vi "GenerationProducerConsumer.vi"() -> ()   [LabVIEW 2022 SP3, in "Generation.lvlib"]
uses:
  Generation.lvlib
  Message.ctl
  FrameProperties.ctl
  <vilib>/platform/TimedLoop/XDataNode/XDataNode.xnode
  <vilib>/Platform/TimedLoop/XDataNode/timing_clust.ctl
  <vilib>/Platform/TimedLoop/XDataNode/XDNodeRunTimeDep.lvlib
  <vilib>/Platform/TimedLoop/XDataNode/wakeup.ctl
  <vilib>/Platform/TimedLoop/XDataNode/nitl_modes.ctl
  <vilib>/DAQmx/write.llb/DAQmx Write (Analog Wfm 1Chan NSamp).vi
panel:
  in  "Cluster":T1={"data"={"t0"=timestamp(0 s since 1904-01-01), "dt"=0.0, "Y"=[]}, "Output task"="", "error in"={"status"=FALSE, "code"=0, "source"=""}}
  in  "queue out":refnum<queue>
  out "task out":refnum<k21>
  out "error out":errorcluster
  out "Generation Duration(ns)":i64
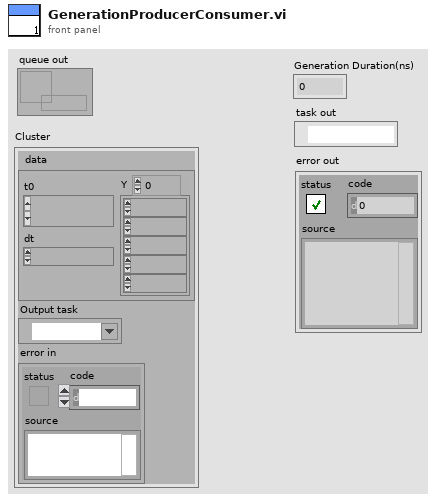
[diagram p1: front panel]
types:
  T1 = cluster{"data":waveform(dbl), "Output task":refnum<k21>, "error in":errorcluster}
  T2 = typedef "XDNodeRunTimeDep.lvlib/timing_clust.ctl" = cluster{"Expected End [f-1]":u64, "Actual End [f-1]":u64, "Finished Late? [f-1]":bool, "Expected End [i-1]":u64, "Actual End [i-1]":u64, "Finished Late? [i-1]":bool, "Expected Start [i]":u64, "Actual Start [i]":u64, "Expected Start [f]":u64, "Actual Start [f]":u64, "Source Name":string, "Structure Name":string, "Period":i64, "Deadline":i64, "Offset":i64, "Start":i64, "Priority":i32, "Timeout":i32, "Mode":T3, "Wakeup Reason":T4, "Error":errorcluster, "Source Type":string, "Secondary Source Type":string, "Global End Time":u64, "Global Start Time":u64, "Frame Duration":u64, "Iteration Duration":u64, "Assigned CPU":i32, "I/O Scan Engine Mode":u32}
  T3 = typedef "XDNodeRunTimeDep.lvlib/nitl_modes.ctl" = enum32{"No Change", "Process missed periods, maintain original phase", "Discard missed periods, maintain original phase", "Process missed periods, ignore original phase", "Discard missed periods, ignore original phase"}
  T4 = typedef "XDNodeRunTimeDep.lvlib/wakeup.ctl" = enum32{"Normal", "Aborted", "Asynchronous wakeup", "Timing source error", "Timed loop error", "Timeout"}
  T5 = typedef "FrameProperties.ctl" = cluster{"Frame Duration":i64, "Actual Start [i]":i64}
  T6 = typedef "Message.ctl" = cluster{"FrameProperties":cluster{"Frame Duration":i64, "Actual Start [i]":i64}, "Data":waveform(dbl), "Identifier":enum16{"Accel", "SignalOut", "ButtonPress"}}
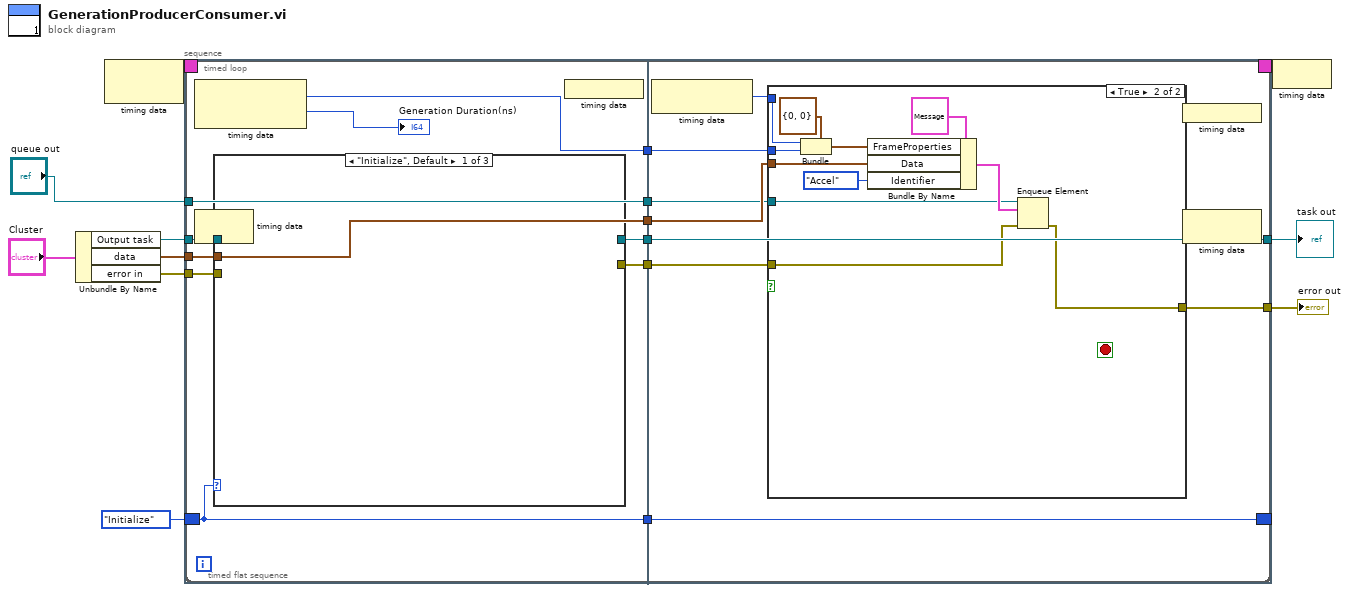
[diagram p0: block diagram]
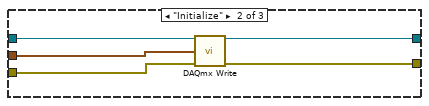
[diagram p2: hidden frame]
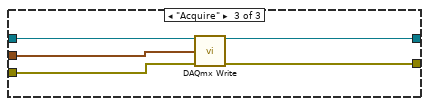
[diagram p3: hidden frame]
diagram:
  n1 = Unbundle By Name("Cluster") -> ("Output task"=w4:refnum<k21>, "data"=w3:waveform(dbl), "error in"=w2:errorcluster)
  n2 = node-c288() -> (w10:T2)  [unwired: 1 in]
  n3 = timed-loop {
    timing: w10 -> [_]
    timing-out: [_] -> w9
    tunnel: w4 -> [w18]
    tunnel: [w17] -> w7
    tunnel: "queue out" -> [w16]
    tunnel: [w15] -> w8
    tunnel: w2 -> [w14]
    tunnel: w3 -> [w13]
    shift-right: [w12] -> _
    shift-left: enum16{"Initialize", "Acquire", "Stop"}."Initialize" -> [w11]
    stop <- _ stop-if-true
    n4 = timed-sequence {
      timing: _ -> [_]
      timing-out: _ -> [_]
      tunnel: w18 -> [w32]
      tunnel: [w26] -> w17
      tunnel: w16 -> [w25]
      tunnel: [w24] -> w15
      tunnel: w14 -> [w23]
      tunnel: w13 -> [w22]
      tunnel: [w20] -> w12
      tunnel: w11 -> [w19]
      n5 = timed-flat-sequence {
        tunnel: w32 -> [w41]
        tunnel: [w39] -> w31
        tunnel: [w34] -> w30
        tunnel: [w38] -> w29
        tunnel: [w37] -> w28
        tunnel: [w36] -> w27
        tunnel: w25 -> [w38]
        tunnel: w23 -> [w35]
        tunnel: w22 -> [w34]
        tunnel: [w33] -> w21
        tunnel: w19 -> [w33]
        tunnel: w31 -> [w62]
        tunnel: w30 -> [w61]
        tunnel: w29 -> [w60]
        tunnel: w28 -> [w59]
        tunnel: w27 -> [w57]
        tunnel: [w57] -> w26
        tunnel: [w58] -> w24
        tunnel: w21 -> [w56]
        tunnel: [w56] -> w20
        frame #0 {
          n6 = node-c288() -> (w39:i64, →"Generation Duration(ns)":i64)  [unwired: 1 in]
          n7 = case shown="\"Initialize\", Default" w33 {
            tunnel: w41 -> [_ w46 w51]
            tunnel: [_ w45 w50] -> w37
            tunnel: [_ w44 w49] -> w36
            tunnel: w35 -> [_ w43 w48]
            tunnel: w34 -> [_ w42 w47]
            frame "Initialize", Default {
            }
            frame "Initialize" {
              n8 = call-poly <vilib>:"DAQmx Write.vi"("task/channels in"=w46, "data"=w42, "error in"=w43) -> ("task out"=w44:refnum<k21>, "error out"=w45:errorcluster)  [unwired: 10 in, 1 out]
            }
            frame "Acquire" {
              n9 = call-poly <vilib>:"DAQmx Write.vi"("task/channels in"=w51, "data"=w47, "error in"=w48) -> ("task out"=w49:refnum<k21>, "error out"=w50:errorcluster)  [unwired: 10 in, 1 out]
            }
          }
          n10 = node-c288() -> ()  [unwired: 1 out]
        }
        frame #1 {
          n11 = node-c288() -> (w63:i64)  [unwired: 1 in]
          n12 = case shown="True" {
            selector: _ -> [_ _]
            tunnel: w63 -> [_ w71]
            tunnel: w62 -> [_ w70]
            tunnel: w61 -> [_ w69]
            tunnel: w60 -> [_ w68]
            tunnel: w59 -> [_ w67]
            tunnel: [_ w66] -> w58
            frame False {
            }
            frame True {
              n13 = Bundle(cluster=T5 {"Frame Duration"=0, "Actual Start [i]"=0} ("FrameProperties"), "Frame Duration"=w71, "Actual Start [i]"=w70) -> (w73:T5)
              n14 = Bundle By Name(cluster=T6 {"FrameProperties"={"Frame Duration"=0, "Actual Start [i]"=0}, "Data"={"t0"=timestamp(0 s since 1904-01-01), "dt"=1.0, "Y"=[]}, "Identifier"=enum."Accel"} ("input cluster"), "FrameProperties"=w73, "Data"=w69, "Identifier"=enum16{"Accel", "SignalOut", "ButtonPress"}."Accel") -> (w74:T6)
              n15 = Enqueue Element(queue=w68, element=w74, error in (no error)=w67) -> (error out=w66:errorcluster)  [unwired: 1 in, 2 out]
            }
          }
          n16 = node-c288() -> ()  [unwired: 1 out]
        }
      }
    }
    n17 = node-c288() -> ()  [unwired: 1 in, 1 out]
    n18 = node-c288() -> ()  [unwired: 1 in, 1 out]
  }
  "error out" <- w8
  "task out" <- w7
  n19 = node-c288(w9) -> ()
